vi "Detect Edge.vi"(10 "Edge Type?":enum16{"Rising", "Falling"}(ring), 11 "Signal In":bool) -> (3 "Edge Detected?":bool)   [LabVIEW 2014]
doc: "This VI takes in a digital signal one point at a time and detects either a rising edge or a falling edge based on the input option specified."
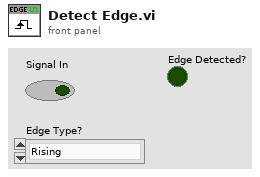
[diagram p1: front panel]
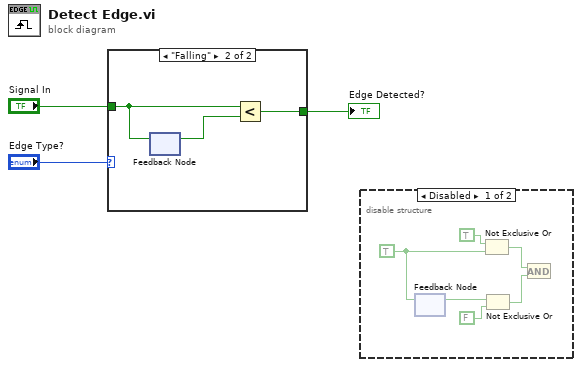
[diagram p0: block diagram]
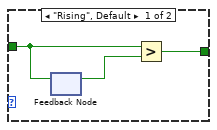
[diagram p3: hidden frame]
diagram:
  n1 = case shown="\"Falling\"" "Edge Type?" {
    tunnel: "Signal In" -> [w6 w9]
    tunnel: [w5 w8] -> w1
    frame "Rising", Default {
      n2 = feedback-in #1(w6) -> ()
      n3 = feedback #1() -> (w4:bool)  [unwired: 1 in]
      n4 = Greater?(x=w6, y=w4) -> (0:w5:bool)
    }
    frame "Falling" {
      n5 = feedback-in #2(w9) -> ()
      n6 = feedback #2() -> (w7:bool)  [unwired: 1 in]
      n7 = Less?(x=w9, y=w7) -> (x < y?=w8:bool)
    }
  }
  "Edge Detected?" <- w1
  n8 = disable-structure shown="Disabled" {
    frame Disabled {
      w10 = TRUE ("x")
      n9 = feedback #3() -> (w15:bool)  [unwired: 1 in]
      n10 = feedback-in #3(w10) -> ()
      n11 = Not Exclusive Or(1:w10, 2:TRUE ("x")) -> (0:w11:bool)
      n12 = Not Exclusive Or(1:FALSE ("y"), 2:w15) -> (0:w12:bool)
      n13 = And(x=w11, y=w12) -> ()  [unwired: 1 out]
    }
    frame Enabled {
    }
  }
